vi "SDCP FTOR Decode.vi"(3 "error in (no error)":errorcluster, 4 "FTOR2 frame":u8[](array[numeric]), 5 "FTOR1 frame":u8[](array[numeric])) -> (0 "error out":errorcluster, 2 "out":T1)   [LabVIEW 2020]
uses:
  Typedefs/SDCP FTOR params.ctl
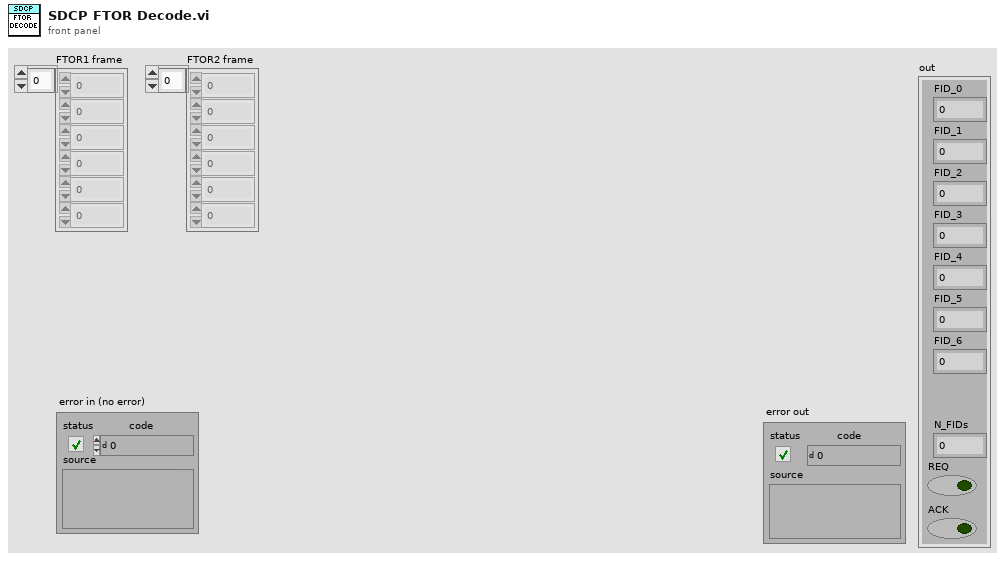
[diagram p1: front panel]
types:
  T1 = typedef "SDCP FTOR params.ctl" = cluster{"FID_0":i32, "FID_1":i32, "FID_2":i32, "FID_3":i32, "FID_4":i32, "FID_5":i32, "FID_6":i32, "N_FIDs":i32, "REQ":bool, "ACK":bool}
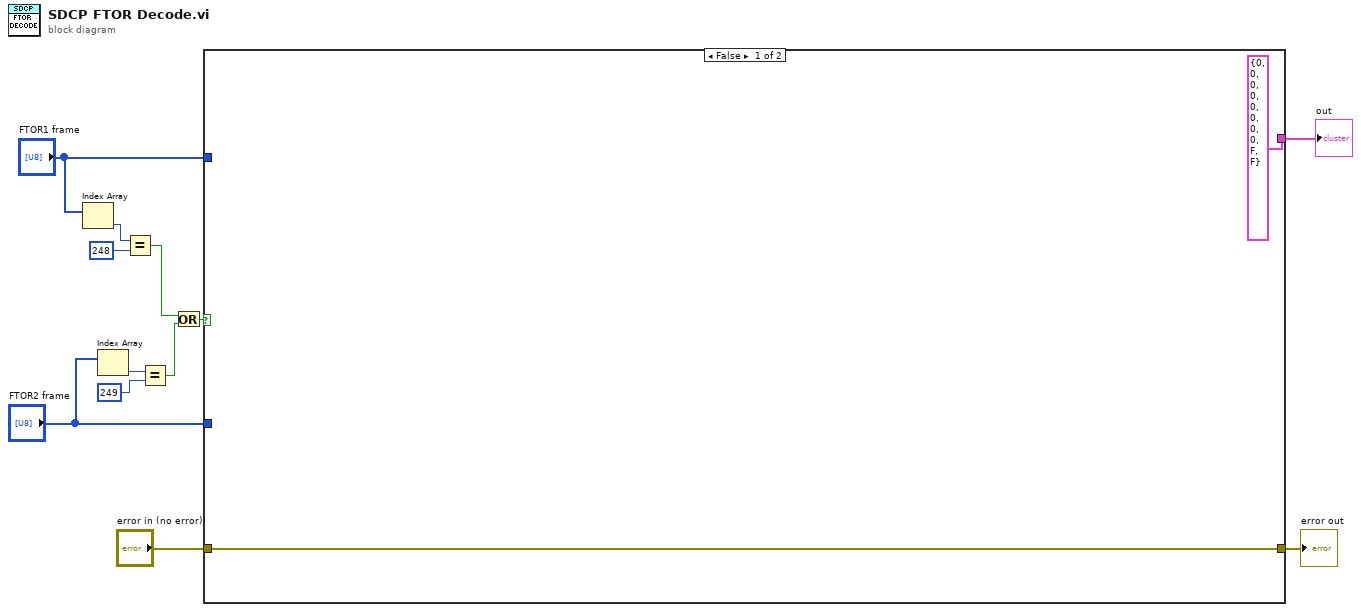
[diagram p0: block diagram]
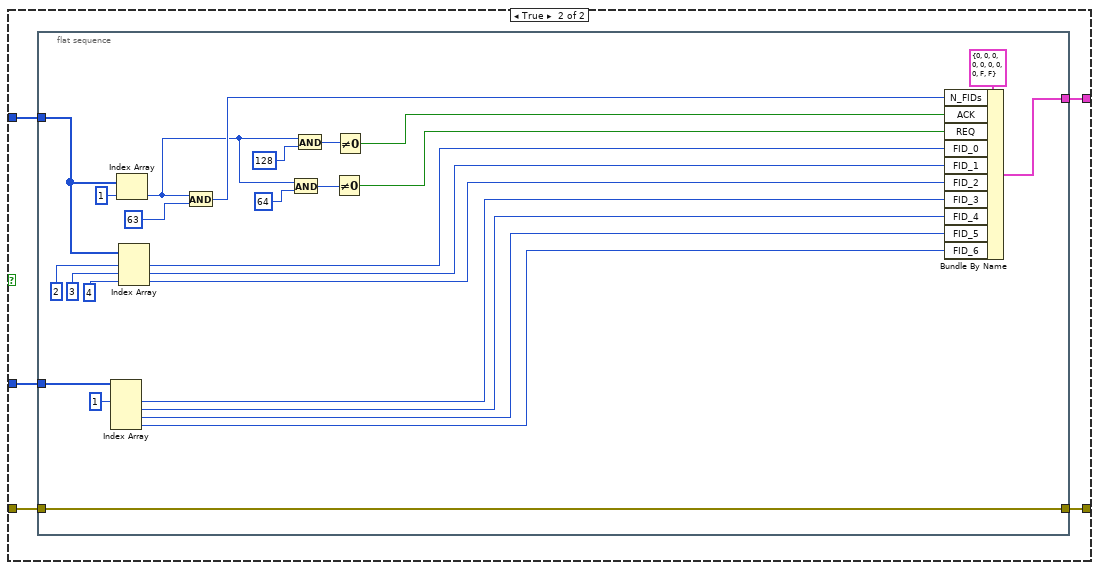
[diagram p2: hidden frame]
diagram:
  n1 = Index Array(array="FTOR1 frame") -> (element=w8:u8)  [unwired: 1 in]
  n2 = Index Array(array="FTOR2 frame") -> (element=w3:u8)  [unwired: 1 in]
  n3 = Equal?(x=w8, y=u8 248) -> (x = y?=w5:bool)
  n4 = Equal?(x=w3, y=u8 249) -> (x = y?=w1:bool)
  n5 = Or(x=w5, y=w1) -> (x .or. y?=w6:bool)
  n6 = case shown="False" w6 {
    tunnel: "error in (no error)" -> [w13 w19]
    tunnel: [w13 w18] -> w11
    tunnel: "FTOR1 frame" -> [_ w17]
    tunnel: "FTOR2 frame" -> [_ w16]
    tunnel: [T1 {"FID_0"=0, "FID_1"=0, "FID_2"=0, "FID_3"=0, "FID_4"=0, "FID_5"=0, "FID_6"=0, "N_FIDs"=0, "REQ"=FALSE, "ACK"=FALSE} ("Cluster") w15] -> w10
    frame False {
    }
    frame True {
      n7 = flat-sequence {
        tunnel: w19 -> [w45]
        tunnel: [w45] -> w18
        tunnel: w17 -> [w33]
        tunnel: w16 -> [w26]
        tunnel: [w41] -> w15
        frame #0 {
          n8 = Index Array(array=w26, index #1=1 ("index")) -> (element #1=w24:u8, element #2=w23:u8, element #3=w22:u8, element #4=w21:u8)  [unwired: 3 in]
          n9 = Index Array(array=w33, index=1) -> (element=w20:u8)
          n10 = Index Array(array=w33, index #1=2 ("index"), index #2=3 ("index"), index #3=4 ("index")) -> (element #1=w29:u8, element #2=w28:u8, element #3=w27:u8)
          n11 = And(x=w20, y=u8 63) -> (x .and. y?=w39:u8)
          n12 = And(x=w20, y=u8 64) -> (x .and. y?=w36:u8)
          n13 = And(x=w20, y=u8 128) -> (x .and. y?=w37:u8)
          n14 = Not Equal To 0?(x=w36) -> (x != 0?=w34:bool)
          n15 = Not Equal To 0?(x=w37) -> (x != 0?=w35:bool)
          n16 = Bundle By Name(cluster=T1 {"FID_0"=0, "FID_1"=0, "FID_2"=0, "FID_3"=0, "FID_4"=0, "FID_5"=0, "FID_6"=0, "N_FIDs"=0, "REQ"=FALSE, "ACK"=FALSE} ("Cluster"), "N_FIDs"=w39, "ACK"=w35, "REQ"=w34, "FID_0"=w29, "FID_1"=w28, "FID_2"=w27, "FID_3"=w24, "FID_4"=w23, "FID_5"=w22, "FID_6"=w21) -> (w41:T1)
        }
      }
    }
  }
  "out" <- w10
  "error out" <- w11
